vi "Read Input Registers.vi"(8 "error in (no error)":errorcluster, 9 "number of input registers":u16, 10 "starting address":u16, 11 "Modbus master in":refnum<class "Modbus Master.lvclass">) -> (0 "error out":errorcluster, 2 "register values":u16[](array[numeric]), 3 "Modbus master out":refnum<class "Modbus Master.lvclass">)   [LabVIEW 2017, in "Modbus Master.lvclass"]
doc: "Reads values from contiguous input registers. The maximum number of input registers this VI can read is 125."
uses:
  <vilib>/Modbus/master/Modbus Master.lvclass
  C:/builds/penguin/iak/lvdsc/trunk/17.0/lv/vi.lib/Modbus/subvis/Modbus API/Modbus API.lvclass
  <vilib>/Modbus/subvis/Modbus API/Modbus API.lvclass/Modbus API.ctl
  <vilib>/Modbus/master/Modbus Master.lvclass/Modbus Master.ctl
  <vilib>/Modbus/subvis/Protocol/Interfaces/Network Master/Network Master.lvclass
  C:/builds/penguin/iak/lvdsc/trunk/17.0/lv/vi.lib/Modbus/subvis/Protocol/Interfaces/Network Protocol/Network Protocol.lvclass
  <vilib>/Modbus/subvis/Transmission Data Unit (ADU)/Transmission Data Unit/Transmission Data Unit.lvclass
  <vilib>/Modbus/subvis/Modbus API/Modbus API.lvclass
  <vilib>/Modbus/subvis/Data and Functions/Master Function Definition/Master Function Definition.lvlib
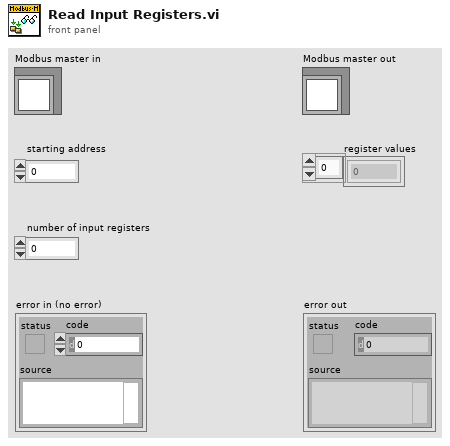
[diagram p1: front panel]
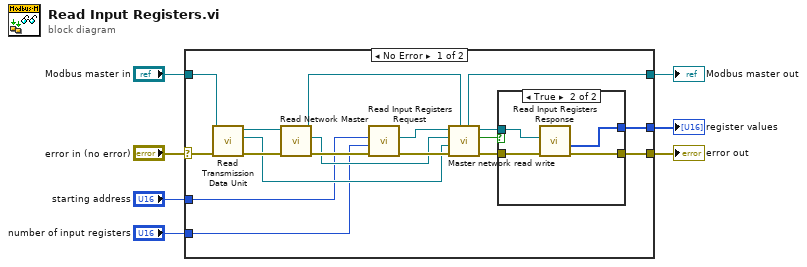
[diagram p0: block diagram]
diagram:
  n1 = case shown="No Error" "error in (no error)" {
    selector: "error in (no error)" -> [w8 w32]
    tunnel: [w19 w32] -> w6
    tunnel: [w13 w31] -> w5
    tunnel: "Modbus master in" -> [w9 w31]
    tunnel: [w14 _] -> w3
    tunnel: "starting address" -> [w12 _]
    tunnel: "number of input registers" -> [w11 _]
    frame No Error {
      n2 = call <vilib>:"Read Transmission Data Unit.vi"("error in (no error)"=w8, "Modbus instance in"=w9) -> ("error out"=w25:errorcluster, "transmission data unit"=w15:refnum<class "Transmission Data Unit.lvclass">, "Modbus instance out"=w24:refnum<class "Modbus Master.lvclass">)  [unwired: 7 in]
      n3 = call <vilib>:"Read Network Master.vi"("error in (no error)"=w25, "Modbus master in"=w24) -> ("error out"=w20:errorcluster, "network master"=w16:refnum<class "Network Master.lvclass">, "Modbus master out"=w21:refnum<class "Modbus Master.lvclass">)  [unwired: 7 in]
      n4 = call <vilib>:"Read Input Registers Request.vi"("error in (no error)"=w20, "number of registers"=w11, "starting address"=w12) -> ("error out"=w22:errorcluster, "Modbus data unit out"=w17:refnum<class "Modbus Data Unit (PDU).lvclass">)  [unwired: 7 in]
      n5 = call <vilib>:"Master network read write.vi"("Modbus master in"=w21, "error in (no error)"=w22, "transmission data unit in"=w15, "network master in"=w16, "Modbus data unit in"=w17) -> ("error out"=w23:errorcluster, "PDU valid?"=w10:bool, "Modbus data unit out"=w18:refnum<class "Modbus Data Unit (PDU).lvclass">, "Modbus master out"=w13:refnum<class "Modbus Master.lvclass">)  [unwired: 3 in]
      n6 = case shown="True" w10 {
        tunnel: w23 -> [w26 w30]
        tunnel: [w26 w29] -> w19
        tunnel: w18 -> [_ w28]
        tunnel: [_ w27] -> w14
        frame False {
        }
        frame True {
          n7 = call <vilib>:"Read Input Registers Response.vi"("error in (no error)"=w30, "Modbus data unit in"=w28) -> ("error out"=w29:errorcluster, "register values"=w27:u16[])  [unwired: 7 in, 1 out]
        }
      }
    }
    frame Error {
    }
  }
  "error out" <- w6
  "Modbus master out" <- w5
  "register values" <- w3
